vi "SpreadsheetRead.vi"() -> (2 "output cluster":cluster{"X Array":dbl[], "Y Array":dbl[]}={"X Array"=[0.0, 0.001, 0.002, 0.003, 0.004, 0.005, 0.006, 0.007, 0.008, 0.009], "Y Array"=[0.0, 1.545, 2.939, 4.045, 4.755, 5.0, 4.755, 4.045, 2.939, 1.545]})   [LabVIEW 2014]
uses:
  <vilib>/Utility/file.llb/Read From Spreadsheet File (DBL).vi
panel:
  out "XY Graph":cluster{"all rows":dbl[], "all rows":dbl[]}(graph)={"all rows"=[0.0, 0.001, 0.002, 0.003, 0.004, 0.005, 0.006, 0.007, 0.008, 0.009], "all rows"=[0.0, 1.545, 2.939, 4.045, 4.755, 5.0, 4.755, 4.045, 2.939, 1.545]}
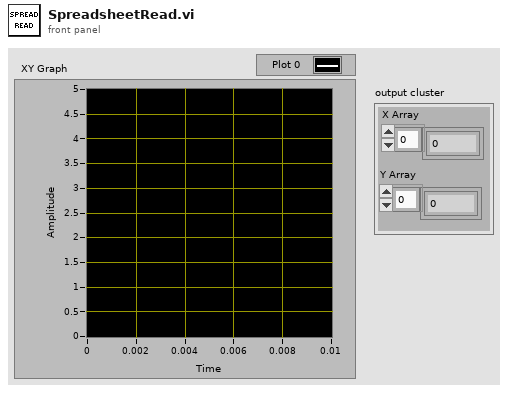
[diagram p1: front panel]
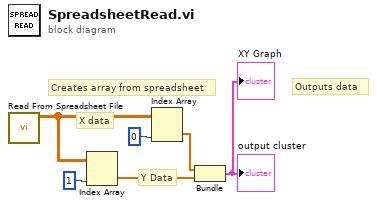
[diagram p0: block diagram]
diagram:
  # "Creates array from spreadsheet"
  # "Outputs data"
  # "Y Data"
  # "X data"
  n1 = call-poly <vilib>:"Read From Spreadsheet File.vi"() -> ("all rows"=w6:dbl[][])  [unwired: 7 in, 4 out]
  n2 = Index Array(array=w6, index (col)=1) -> (element=w2:dbl[])  [unwired: 1 in]
  n3 = Index Array(array=w6, index (col)=0) -> (element=w3:dbl[])  [unwired: 1 in]
  n4 = Bundle("all rows"=w3, "all rows"=w2) -> (→"XY Graph" →"output cluster":cluster{"all rows":dbl[], "all rows":dbl[]})  [unwired: 1 in]
